vi "dPWM_PanelSim_Global.vi"(0 "Menu":T4=enum."delete", 5 "DIO Channel":T1=enum."DIO 1", 7 "Boolean Value":bool, 9 "Numeric Value":dbl format="%#.4f", 11 "error in (no error)":errorcluster, 12 "String Value":string) -> (10 "Value out":T2={"type"="AI", "device"="", "name"="", "data"={"<init"=FALSE, "<duty_cycle"=0.0, "<dio_pin"=0.0}}, 15 "error out":errorcluster)   [LabVIEW 2019]
doc: "This is used to set and get the last motor output values. This is needed for simulation, since we cannot read these values from the hardware.\n\nThis software is licensed. Open the labview\\readme\\WPI Robotics Library Open Source License.txt file for more information."
uses:
  dPWM Data proto.ctl
  dPWM proto.ctl
  dPWM Update Ops.ctl
  <vilib>/Rock Robotics/SystemInterfaces/DIO/FPGA_DIOChannel.ctl
panel:
  out "All Values":T2[](array[typedef])
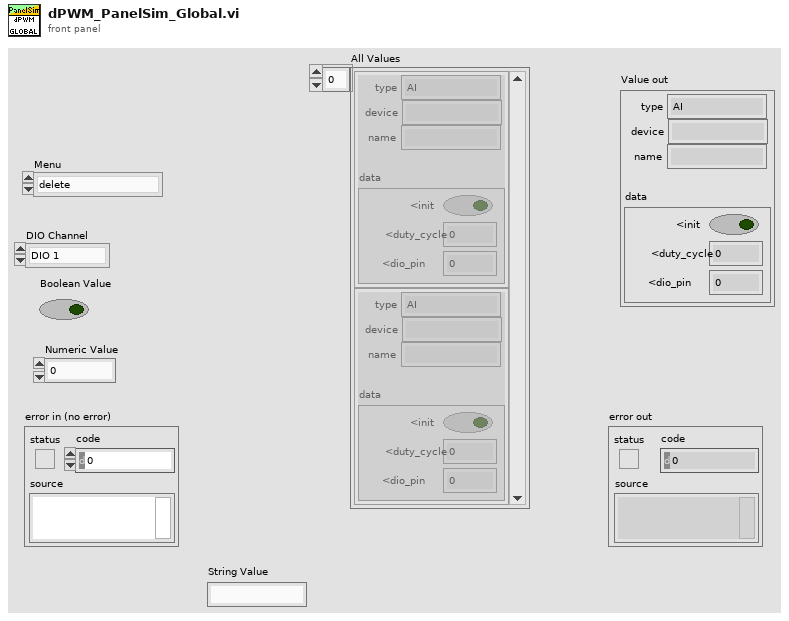
[diagram p1: front panel]
types:
  T1 = typedef "FPGA_DIOChannel.ctl" = enum8{"DIO 0", "DIO 1", "DIO 2", "DIO 3", "DIO 4", "DIO 5", "DIO 6", "DIO 7", "DIO 8", "DIO 9", "DIO MXP 0", "DIO MXP 1", "DIO MXP 2", "DIO MXP 3", "DIO MXP 4", "DIO MXP 5", "DIO MXP 6", "DIO MXP 7", "DIO MXP 8", "DIO MXP 9", "DIO MXP 10", "DIO MXP 11", "DIO MXP 12", "DIO MXP 13", "DIO MXP 14", "DIO MXP 15", "SPI Port CS1", "SPI Port CS2", "SPI Port CS3", "SPI Port MISO", "SPI Port MOSI", "Invalid"}
  T2 = typedef "dPWM proto.ctl" = cluster{"type":string, "device":string, "name":string, "data":T3}
  T3 = typedef "dPWM Data proto.ctl" = cluster{"<init":bool, "<duty_cycle":dbl, "<dio_pin":dbl}
  T4 = typedef "dPWM Update Ops.ctl" = enum16{"get", "delete", "JSON update", "set  name", "transmit initial", "reset", "set init", "set duty cycle", "set dio channel"}
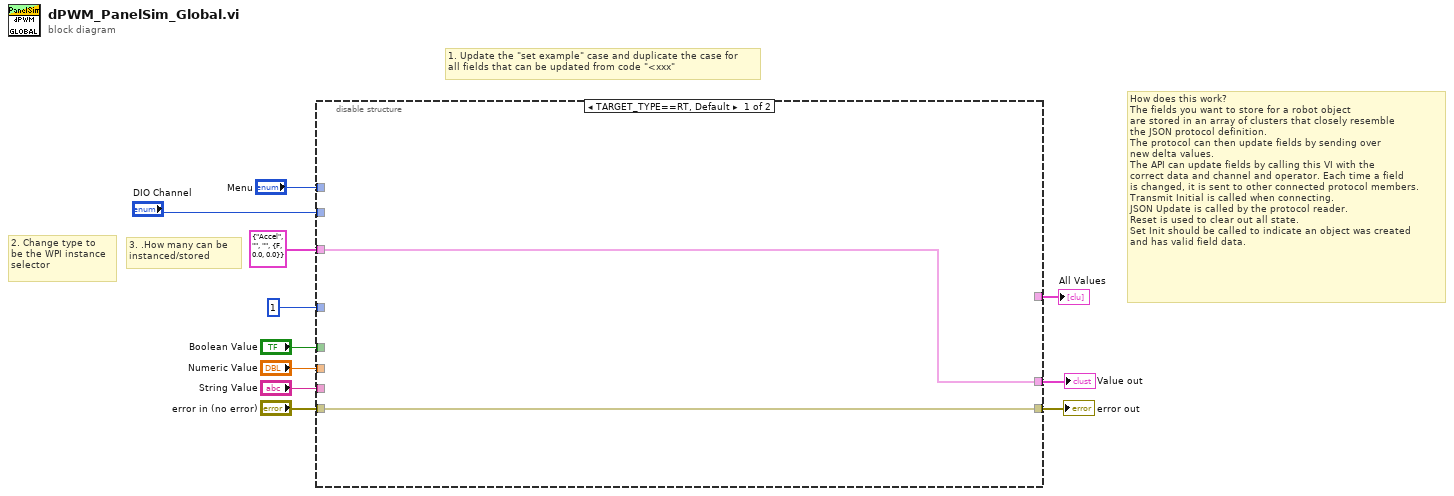
[diagram p0: block diagram]
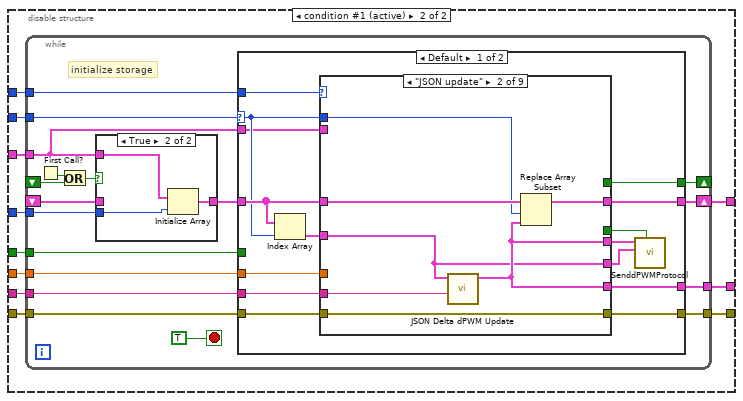
[diagram p2: hidden frame]
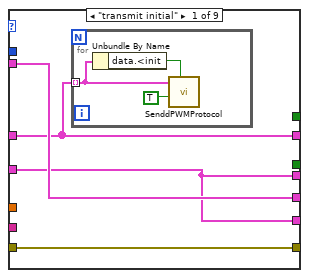
[diagram p3: hidden frame]
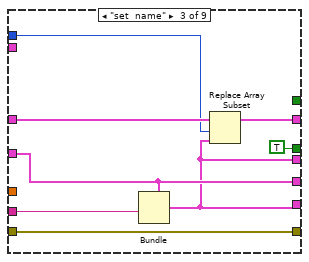
[diagram p4: hidden frame]
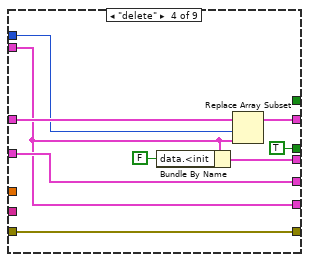
[diagram p5: hidden frame]
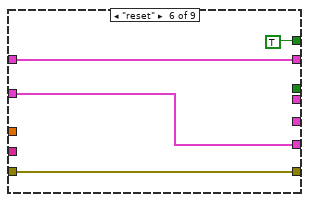
[diagram p7: hidden frame]
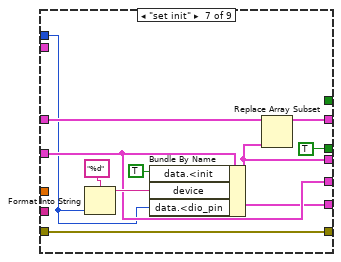
[diagram p8: hidden frame]
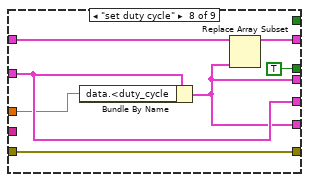
[diagram p9: hidden frame]
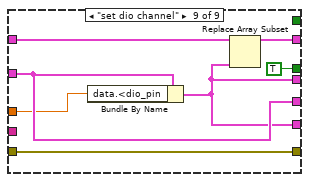
[diagram p10: hidden frame]
diagram:
  # "How does this work?\nThe fields you want to store for a robot object\nare stored in an array of clusters that closely resemble\nthe JSON protocol definition.\nThe protocol can then update fields by sending over\nnew delta values.\nThe API can update fields by calling this VI with the\ncorrect data and channel and operator. Each time a field\nis changed, it is sent to other connected protocol members.\nTransmit Initial is called when connecting.\nJSON Update is called by the protocol reader.\nReset is used to clear out all state.\nSet Init should be called to indicate an object was created\nand has valid field data."
  # "1. Update the \"set example\" case and duplicate the case for\nall fields that can be updated from code \"<xxx\""
  # "2. Change type to\nbe the WPI instance\nselector"
  # "3. .How many can be\ninstanced/stored"
  n1 = disable-structure shown="TARGET_TYPE==RT, Default" {
    disable-tunnel: "Menu" -> [_ w24]
    disable-tunnel: [w13 w23] -> w10
    disable-tunnel: "error in (no error)" -> [w13 w22]
    disable-tunnel: [_ w21] -> w8
    disable-tunnel: "Numeric Value" -> [_ w20]
    disable-tunnel: "DIO Channel" -> [_ w19]
    disable-tunnel: [w12 w18] -> w5
    disable-tunnel: T2 {"type"="Accel", "device"="", "name"="", "data"={"<init"=FALSE, "<duty_cycle"=0.0, "<dio_pin"=0.0}} ("Accel value out") -> [w12 w17]
    disable-tunnel: "String Value" -> [_ w16]
    disable-tunnel: 1 -> [_ w15]
    disable-tunnel: "Boolean Value" -> [_ w14]
    frame condition #0 {
    }
    frame condition #1 (active) {
      n2 = while {
        tunnel: w20 -> [w42]
        tunnel: w22 -> [w38]
        shift-right: [w41] -> w21
        shift-left: _ -> [w34]
        tunnel: [w40] -> w18
        tunnel: w24 -> [w39]
        tunnel: [w37] -> w23
        tunnel: w19 -> [w33]
        tunnel: w17 -> [w32]
        tunnel: w16 -> [w31]
        shift-right: [w27] -> _
        shift-left: _ -> [w28]
        tunnel: w15 -> [w26]
        tunnel: w14 -> [w25]
        stop <- TRUE stop-if-true
        # "initialize storage"
        n3 = First Call?() -> (First Call?: T/F=w29:bool)
        n4 = Or(x=w29, y=w28) -> (x .or. y?=w30:bool)
        n5 = case shown="True" w30 {
          tunnel: [w123 w126] -> w35
          tunnel: w34 -> [w123 _]
          tunnel: w32 -> [_ w125]
          tunnel: w26 -> [_ w124]
          frame False {
          }
          frame True {
            n6 = Initialize Array(w125, w124) -> (w126:T2[])
          }
        }
        n7 = case shown="Default" w33 {
          selector: w33 -> [w50 _]
          tunnel: w42 -> [w57 _]
          tunnel: [w56 w122] -> w41
          tunnel: [w55 w120] -> w40
          tunnel: w39 -> [w54 _]
          tunnel: w38 -> [w53 w121]
          tunnel: [w52 w121] -> w37
          tunnel: w35 -> [w51 w122]
          tunnel: w32 -> [w48 w120]
          tunnel: w31 -> [w47 _]
          tunnel: [w46 _] -> w27
          tunnel: w25 -> [_ _]
          frame Default {
            n8 = Index Array(array=w51, index=w50) -> (element=w49:T2)
            n9 = case shown="\"JSON update\"" w54 {
              tunnel: w57 -> [_ _ _ _ _ _ _ w106 w113]
              tunnel: [w58 w71 w79 w87 w91 w95 w101 w111 w118] -> w56
              tunnel: w51 -> [w58 w69 w77 w88 w91 w95 w100 w110 w117]
              tunnel: [w59 w67 w72 w81 w89 w93 w98 w108 w115] -> w55
              tunnel: [w61 w70 w78 w86 w90 w94 w97 w107 w114] -> w52
              tunnel: w53 -> [w61 w70 w78 w86 w90 w94 w97 w107 w114]
              tunnel: w50 -> [_ w68 w75 w83 _ _ w96 _ _]
              tunnel: [w59 w67 w72 w82 _ _ w98 w108 w115] -> w44
              tunnel: [w60 w65 w74 w84 _ _ w99 w109 w116] -> w43
              tunnel: [_ _ TRUE TRUE _ _ TRUE TRUE TRUE] -> w45
              tunnel: w49 -> [w59 w65 w74 w84 w89 w93 w99 w109 w116]
              tunnel: w48 -> [w60 _ _ w81 _ _ _ _ _]
              tunnel: w47 -> [_ w66 w73 _ _ _ _ _ _]
              tunnel: [_ _ _ _ _ TRUE _ _ _] -> w46
              frame "transmit initial" {
                n10 = for {
                  tunnel: w58 -> [w63] mode=indexing
                  n11 = Unbundle By Name(w63) -> ("data.<init"=w64:bool)
                  n12 = call "SenddPWMProtocol.vi"("Send"=w64, "Initialize"=TRUE ("Send"), "Tmpl values"=w63) -> ()  [unwired: 9 in]
                }
              }
              frame "JSON update" {
                n13 = call "JSON Delta dPWM Update.vi"("Delta JSON"=w66, "Tmpl values"=w65) -> ("Tmpl values"=w67:T2)  [unwired: 8 in, 1 out]
                n14 = Replace Array Subset(array=w69, new element=w67, index=w68) -> (w71:T2[])
              }
              frame "set  name" {
                n15 = Bundle(cluster=w74, "name"=w73) -> (w72:T2)  [unwired: 3 in]
                n16 = Replace Array Subset(array=w77, new element=w72, index=w75) -> (w79:T2[])
              }
              frame "delete" {
                n17 = Bundle By Name(cluster=w81, "data.<init"=FALSE) -> (w82:T2)
                n18 = Replace Array Subset(array=w88, new element=w81, index=w83) -> (w87:T2[])
              }
              frame "get" {
              }
              frame "reset" {
              }
              frame "set init" {
                n19 = Format Into String(format string="%d", w96) -> (resulting string=w103:string)  [unwired: 2 in, 1 out]
                n20 = Bundle By Name(cluster=w99, "data.<init"=TRUE, "device"=w103, "data.<dio_pin"=w96) -> (w98:T2)
                n21 = Replace Array Subset(array=w100, new element=w98) -> (w101:T2[])  [unwired: 1 in]
              }
              frame "set duty cycle" {
                n22 = Bundle By Name(cluster=w109, "data.<duty_cycle"=w106) -> (w108:T2)
                n23 = Replace Array Subset(array=w110, new element=w108) -> (w111:T2[])  [unwired: 1 in]
              }
              frame "set dio channel" {
                n24 = Bundle By Name(cluster=w116, "data.<dio_pin"=w113) -> (w115:T2)
                n25 = Replace Array Subset(array=w117, new element=w115) -> (w118:T2[])  [unwired: 1 in]
              }
            }
            n26 = call "SenddPWMProtocol.vi"("Send"=w45, 10:"Tmpl values"=w43, 11:"Tmpl values"=w44) -> ()  [unwired: 9 in]
          }
          frame "Invalid" {
            # "Do nothing if \nchannel is Invalid."
          }
        }
      }
    }
  }
  "error out" <- w10
  "Value out" <- w5
  "All Values" <- w8
